vi "Filter Check.vi"(8 "Pattern without asterisk":string[](array[string]), 11 "path":path) -> (3 "Include Info":bool)   [LabVIEW 2020, in "SimpleDependencyInspector.lvlib"]
uses:
  SimpleDependencyInspector.lvlib
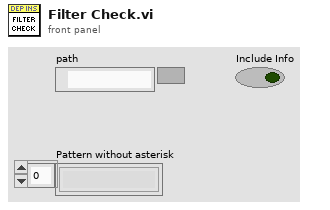
[diagram p1: front panel]
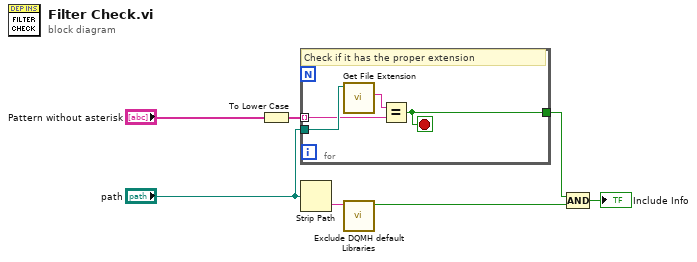
[diagram p0: block diagram]
diagram:
  n1 = To Lower Case(string="Pattern without asterisk") -> (all lower case string=w4:string[])
  n2 = for {
    tunnel: "path" -> [w11]
    tunnel: w4 -> [w10] mode=indexing
    tunnel: [w9] -> w5
    stop <- w9 stop-if-true
    # "Check if it has the proper extension"
    n3 = call <vilib>:"Get File Extension.vi"("file"=w11) -> ("lowercase file extension"=w8:string)  [unwired: 6 in, 4 out]
    n4 = Equal?(x=w8, y=w10) -> (x = y?=w9:bool)
  }
  n5 = Strip Path(path="path") -> (name=w1:string)  [unwired: 1 out]
  n6 = call "Exclude DQMH default Libraries.vi"("name"=w1) -> ("Is not a DQMH Default Lib?"=w3:bool)  [unwired: 10 in]
  n7 = Compound Arithmetic op=AND(w5, w3) -> (→"Include Info":bool)
